vi "Material-ConfigPage-ReadyForSubPanel.vi"(0 "Configuration Page":refnum<class "Material-ConfigPage.lvclass">, 11 "error in":errorcluster) -> (4 "Configuration Page out":refnum<class "Material-ConfigPage.lvclass">, 15 "error out":errorcluster)   [LabVIEW 2013, in "Material-ConfigPage.lvclass"]
uses:
  Material-ConfigPage.lvclass
  Material-ConfigPage.lvclass/Material-ConfigPage.ctl
panel:
  # "Inputs"
  # "Outputs"
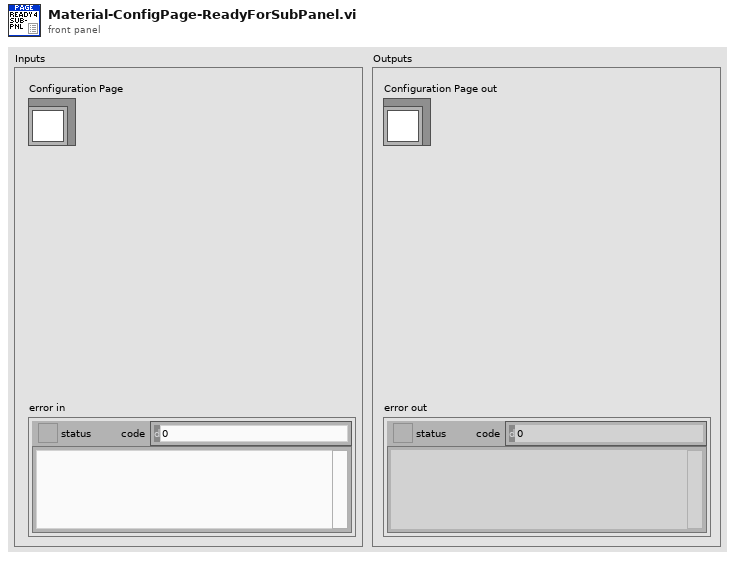
[diagram p1: front panel]
types:
  T1 = cluster{"PageID":string, "vi reference":refnum<vi>}
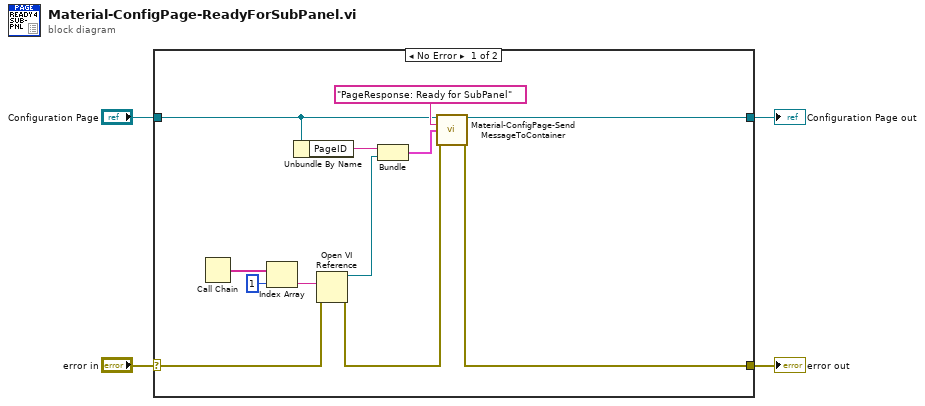
[diagram p0: block diagram]
diagram:
  n1 = case shown="No Error" "error in" {
    selector: "error in" -> [w10 w18]
    tunnel: [w14 w18] -> w4
    tunnel: [w16 w17] -> w2
    tunnel: "Configuration Page" -> [w8 w17]
    frame No Error {
      n2 = Call Chain() -> (call chain=w13:string[])
      n3 = Index Array(array=w13, index=1) -> (element=w11:string)
      n4 = Unbundle By Name(w8) -> ("PageID"=w7:string)
      n5 = Open VI Reference(vi path=w11, error in (no error)=w10) -> (vi reference=w5:refnum<vi>, error out=w9:errorcluster)  [unwired: 4 in]
      n6 = Bundle("PageID"=w7, "vi reference"=w5) -> (w6:T1)  [unwired: 1 in]
      n7 = call "Material-ConfigPage-SendMessageToContainer.vi"("Configuration Page"=w8, "Parameter"="PageResponse: Ready for SubPanel", "Payload"=w6, "error in"=w9) -> ("Configuration Page out"=w16:refnum<class "Material-ConfigPage.lvclass">, "error out"=w14:errorcluster)  [unwired: 10 in]
    }
    frame Error {
    }
  }
  "error out" <- w4
  "Configuration Page out" <- w2
